vi "BonOMM-SAOMM.vi"() -> ()   [LabVIEW 2019] (continued)
                          frame False {
                            w3634 = i16 0 items=["tel coords", "tel offset", "guidage"] ("options")
                            n5502 = local read "Obslib"() -> (w3635:string[][])
                            n5503 = Build Array(w3632, w3631, w3630, w3629) -> (w3636:string[])
                            n5504 = call "Coords to chart(new).vi"("DataLine"=w3636, "options"=w3634, "Tableau entrant"=w3635) -> ("historique"=w3637:string[][])
                            n5505 = local write "Obslib"(w3637) -> ()
                          }
                          frame True {
                            w3643 = i16 0 items=["tel coords", "tel offset", "guidage"] ("options")
                            n5506 = local read "Obslib"() -> (w3644:string[][])
                            n5507 = Build Array(w3639, w3640, w3641, w3638) -> (w3645:string[])
                            n5508 = call "Coords to chart(new).vi"("DataLine"=w3645, "options"=w3643, "Tableau entrant"=w3644) -> ("historique"=w3646:string[][])
                            n5509 = local write "Obslib"(w3646) -> ()
                          }
                        }
                        "From library" <- w3626
                        n5510 = Number To Fractional String(number=w3599, width (-)=i16 4, precision (6)=w3619) -> (F-format string=w3612:string)  [unwired: 1 in]
                        n5511 = Number To Fractional String(number=w3598, width (-)=w3618, precision (6)=w3619) -> (F-format string=w3617:string)  [unwired: 1 in]
                        n5512 = Number To Fractional String(number=w3597, width (-)=w3618, precision (6)=w3619) -> (F-format string=w3616:string)  [unwired: 1 in]
                        n5513 = Search and Replace String(replace all?=w3613, input string=w3617, search string=w3614, replace string=w3615) -> (result string=w3611:string)  [unwired: 4 in, 3 out]
                        n5514 = Search and Replace String(replace all?=w3613, input string=w3616, search string=w3614, replace string=w3615) -> (result string=w3610:string)  [unwired: 4 in, 3 out]
                        n5515 = local read "path_pointing"() -> (w3609:path)
                        n5516 = Concatenate Strings(w3612, w3607, w3611, w3607, w3610, ".pnt") -> (w3608:string)
                        n5517 = Build Path(base path=w3609, name or relative path=w3608) -> (appended path=w3594:path)
                        n5518 = local read "File I/O Error"() -> (w3596:errorcluster)
                        n5519 = call "PNT-Data-Write.vi"("Path IN"=w3594, "Data Line"=w3593, "Error IN"=w3596) -> ("Error OUT"=w3595:errorcluster)  [unwired: 11 in, 1 out]
                        n5520 = local write "File I/O Error"(w3595) -> ()
                      }
                    }
                  }
                  frame True {
                    w3647 = 2
                    # "Début d'un déplacement"
                    # "Désactiver les boutons de TCS"
                    n5521 = property on="GO" class="Bool (strict)"("Disabled"=w3647) -> ()  [unwired: 2 in, 2 out]
                    n5522 = property on="ModifFoyer" class="Bool (strict)"("Disabled"=w3647) -> ()  [unwired: 2 in, 2 out]
                    n5523 = property on="Écran" class="Bool (strict)"("Disabled"=w3647) -> ()  [unwired: 2 in, 2 out]
                    n5524 = property on="ModCoor" class="Bool (strict)"("Disabled"=w3647) -> ()  [unwired: 2 in, 2 out]
                    n5525 = property on="Zénith" class="Bool (strict)"("Disabled"=w3647) -> ()  [unwired: 2 in, 2 out]
                    n5526 = property on="Range" class="Bool (strict)"("Disabled"=w3647) -> ()  [unwired: 2 in, 2 out]
                    n5527 = property on="Synctel" class="Bool (strict)"("Disabled"=w3647) -> ()  [unwired: 2 in, 2 out]
                    n5528 = property on="ModifRotation" class="Bool (strict)"("Disabled"=w3647) -> ()  [unwired: 2 in, 2 out]
                    n5529 = property on="Offset OK" class="Bool (strict)"("Disabled"=w3647) -> ()  [unwired: 2 in, 2 out]
                    n5530 = property on="ModifDome" class="Bool (strict)"("Disabled"=w3647) -> ()  [unwired: 2 in, 2 out]
                  }
                }
              }
            }
            n5531 = local read "Quit"() -> (w3405:bool)
          }
          "Événements Software" <- w978
          n5532 = while {
            tunnel: [w1297] -> w976
            stop <- w1297 stop-if-true
            # "Boucle périodique pour PrAMS + Hexapode + LVDTs\nÉvénements lents ..."
            n5533 = stacked-sequence {
              frame #0 {
                n5534 = disable-structure shown="Disabled" {
                  frame Disabled {
                    n5535 = local read "LVDT-RA"() -> (w1301:refnum<k21>)
                    n5536 = local read "LVDT Error"() -> (w1300:errorcluster)
                    n5537 = Unbundle By Name(w1300) -> ("status"=w1299:bool)
                    n5538 = case shown="Faux" w1299 {
                      tunnel: w1301 -> [w1314 _]
                      tunnel: w1300 -> [_ _]
                      frame False {
                        n5539 = call "Read-LVDT-Data.vi"("shared variable refnum"=w1314, "MaxLen"=631 ("timeout ms"), "Data IN"="LVDT-RA-Data") -> ("Graph Data"=w1308:dbl[], "Data OUT"=w1310:dbl[], "error out"=→"LVDT Error":errorcluster)  [unwired: 10 in]
                        "Graph Data" <- w1308
                        n5540 = local write "LVDT-RA-Data"(w1310) -> ()
                        n5541 = Subtract(x=w1308, y="LVDT-zero") -> (x-y=w1315:dbl[])
                        n5542 = Multiply(x="LVDT-scale", y=w1315) -> (x*y=w1305:dbl[])
                        n5543 = Array Size(array=w1305) -> (size(s)=w1304:i32)
                        n5544 = Decrement(x=w1304) -> (x-1=w1302:i32)
                        n5545 = Bundle(0.0, "LVDT-time"="LVDT-time", w1305) -> (→"LVDT-RA-coarse" →"LVDT-RA-closeup":cluster{dbl, "LVDT-time":dbl, dbl[]})  [unwired: 1 in]
                        n5546 = Index Array(array=w1305, index=w1302) -> (element=→"LVDT-RA-inst":dbl)
                      }
                      frame True {
                      }
                    }
                  }
                  frame Enabled {
                  }
                }
              }
              frame #1 {
                # "Si la communication avec TCS et PrAMS sont actives, on update les valeurs de ALT/AZ/ROT de Prams\n\nN.B. : L'erreur associée (#64) : est ignorée par la boucle \"emterror\" ci-bas ..."
                n5547 = local read "PrAMS COMM"() -> (w1319:bool)
                n5548 = local read "TCS COMM"() -> (w1320:bool)
                n5549 = And(x=w1320, y=w1319) -> (x .and. y?=w1318:bool)
                n5550 = case shown="Faux" w1318 {
                  frame False {
                  }
                  frame True {
                    n5551 = local read "Epoch Tel"() -> (w1334:dbl)
                    n5552 = local read "RA Tel"() -> (w1338:dbl)
                    n5553 = local read "DEC Tel"() -> (w1337:dbl)
                    n5554 = local read "AnnéeRL"() -> (w1333:dbl)
                    n5555 = local read "LST"() -> (w1332:dbl)
                    n5556 = call "ad2deg.vi"("DEC (sec)"=w1337, "RA (sec)"=w1338) -> ("DEC (°)"=w1335:dbl, "RA (°)"=w1336:dbl)
                    n5557 = call "ad2deg.vi"("RA (sec)"=w1332) -> ("RA (°)"=w1331:dbl)  [unwired: 1 in, 1 out]
                    n5558 = call "precess.vi"("Eq2"=w1333, "Eq1"=w1334, "DEC 1"=w1335, "RA 1"=w1336) -> ("DEC 2"=w1329:dbl, "RA 2"=w1339:dbl)
                    "DEC" <- w1329
                    n5559 = Subtract(x=w1331, y=w1339) -> (x-y=w1330:dbl)
                    "HA" <- w1330
                    n5560 = control-ref of="PrAMS-ACK"() -> (w1324:refnum<vi>)
                    n5561 = control-ref of="PrAMS actif"() -> (w1323:refnum<vi>)
                    n5562 = local read "PrAMS VRN"() -> (w1325:refnum<visa-resource-name>)
                    n5563 = local read "PrAMS Error"() -> (w1326:errorcluster)
                    n5564 = local read "Signature"() -> (w1328:u32)
                    n5565 = local read "MessageType"() -> (w1327:cluster{string[], u32[]})
                    n5566 = call "SAOMM-SetTelescopeProperties.vi"("PRAMMS-COMM IN"=w1325, "PramsActif"=w1323, "PrAMS-ACK"=w1324, "HA"=w1330, "DEC"=w1329, "Error IN"=w1326, "Signature"=w1328, "MsgTypeEnum"=w1327) -> ("PRAMMS-COMM OUT"=w1321:refnum<visa-resource-name>, "Error OUT"=w1322:errorcluster)  [unwired: 6 in]
                    n5567 = local write "PrAMS VRN"(w1321) -> ()
                    n5568 = local write "PrAMS Error"(w1322) -> ()
                  }
                }
              }
              frame #2 {
                # "L'angle ne peut être envoyé que si l'asservissement est OFF"
                n5569 = local read "Servo"() -> (w1340:bool)
                n5570 = case shown="Faux" w1340 {
                  frame False {
                    # "Prams à un 180° dans sa matrice d'Euler"
                    n5571 = local read "RotationEffective"() -> (w1351:dbl)
                    n5572 = control-ref of="PrAMS-ACK"() -> (w1343:refnum<vi>)
                    n5573 = local read "PrAMS VRN"() -> (w1346:refnum<visa-resource-name>)
                    n5574 = local read "PrAMS Error"() -> (w1347:errorcluster)
                    n5575 = local read "MessageType"() -> (w1348:cluster{string[], u32[]})
                    n5576 = control-ref of="PrAMS actif"() -> (w1344:refnum<vi>)
                    n5577 = local read "Signature"() -> (w1345:u32)
                    n5578 = call "Fix_angle.vi"("±180 -> 0-360?"=FALSE, "Angle IN"=w1351) -> ("Angle OUT"=w1350:dbl)  [unwired: 3 in]
                    n5579 = Negate(x=w1350) -> (-x=w1341:dbl)
                    n5580 = call-poly "SAOMM-Num2littleEndian.vi"("Number"=w1341) -> ("LiitleEndianedData"=w1349:u8[])  [unwired: 14 in]
                    n5581 = call "SAOMM-SendSET.vi"("PRAMMS-COMM IN"=w1346, "Active Refnum"=w1344, "PrAMS-ACK"=w1343, "Signature"=w1345, "Error IN"=w1347, "MessageType"=w1348, "Active SET"="emtSetMountingPlateAngle", "Value (little endianed byte array)"=w1349) -> ()  [unwired: 4 in, 4 out]
                  }
                  frame True {
                  }
                }
              }
              frame #3 {
                # "Enregistre environ 2 fois par \"Considered Lenght\""
                # "Update l'historique de guidage et enregistre log dans un fichier ..."
                n5582 = local read "Graph-Centroids"() -> (w1355:cluster{"TimeArray":dbl[], dbl[]}[])
                n5583 = Index Array(array=w1355) -> (element #1=w1372:cluster{"TimeArray":dbl[], dbl[]}, element #2=w1371:cluster{"TimeArray":dbl[], dbl[]})  [unwired: 2 in]
                n5584 = Unbundle(w1372) -> (w1369:dbl[])  [unwired: 1 out]
                n5585 = Unbundle(w1371) -> ("TimeArray"=w1354:dbl[], w1370:dbl[])
                n5586 = local read "LastSaveTimeStamp"() -> (w1361:dbl)
                n5587 = local read "ConsideredLenght"() -> (w1365:i32)
                n5588 = call "TimeStamp-Extractor.vi"("TimeStampArray"=w1354) -> ("LastTimestamp"=w1360:dbl)  [unwired: 12 in, 2 out]
                n5589 = To Double Precision Float(number=w1365) -> (double precision float=w1364:dbl)
                n5590 = call "Guide_error_histo.vi"("X Array"=w1369, "intervals"=11, "Y array"=w1370, "limite haute"=5.0, "limite basse"=-5.0 ("limite haute")) -> ("XY graph"=→"Guiderreur":cluster{dbl[], dbl[]}[])  [unwired: 1 out]
                n5591 = local read "CentroidsData"() -> (w1356:cluster{dbl[], dbl[]}[])
                n5592 = expression code="x/2"(w1364) -> (w1363:dbl)
                n5593 = Add(x=w1361, y=w1363) -> (x+y=w1362:dbl)
                n5594 = Greater?(x=w1360, y=w1362) -> (0:w1358:bool)
                n5595 = Or(x="ForceSaveToFile", y=w1358) -> (x .or. y?=w1359:bool)
                n5596 = case shown="Vrai" w1359 {
                  tunnel: w1360 -> [_ w1399]
                  tunnel: w1361 -> [_ w1384]
                  tunnel: w1356 -> [_ w1400]
                  frame False {
                  }
                  frame True {
                    # "Va peut-être perdre les quelques minutes juste avant la fermeture \n... pour ce que ça changera c'est beaucoup de travail."
                    n5597 = local read "path_trackfile"() -> (w1383:path)
                    n5598 = Strip Path(path=w1383) -> (stripped path=w1377:path)  [unwired: 1 out]
                    n5599 = local read "path_trackfile"() -> (w1397:path)
                    n5600 = Build Path(base path=w1377, name or relative path="Hexapod") -> (appended path=w1375:path)
                    n5601 = call "GetPathFromTimeStamp.vi"("UTC Time"=FALSE, "LocalTimeStamp"=w1384, "Changement de date à midi ?"=TRUE) -> ("Date String"=w1373:string)  [unwired: 11 in, 1 out]
                    n5602 = call "CheckAndCreateDirectory.vi"("Path IN"=w1375) -> ("Path OUT"=w1374:path, "Exists?"=w1380:bool, "Created?"=w1379:bool)  [unwired: 12 in]
                    n5603 = call "GetPathFromTimeStamp.vi"("UTC Time"=TRUE, "LocalTimeStamp"=w1399, "Changement de date à midi ?"=TRUE) -> ("Date String"=w1398:string)  [unwired: 11 in, 1 out]
                    n5604 = local read "ForceSaveToFile"() -> (w1389:bool)
                    n5605 = Build Path(base path=w1397, name or relative path=w1398) -> (appended path=w1396:path)
                    n5606 = Or(x=w1380, y=w1379) -> (x .or. y?=w1378:bool)
                    n5607 = local read "Servo"() -> (w1388:bool)
                    n5608 = case shown="Vrai" w1378 {
                      tunnel: w1384 -> [_ w1407]
                      tunnel: w1374 -> [_ w1406]
                      tunnel: w1373 -> [_ w1404]
                      frame False {
                      }
                      frame True {
                        # "Log de l'hexapode"
                        n5609 = Concatenate Strings(w1404, ".hex") -> (w1402:string)
                        n5610 = local read "HexXData"() -> (w1409:cluster{dbl[], dbl[]}[])
                        n5611 = local read "HexYData"() -> (w1408:cluster{dbl[], dbl[]}[])
                        n5612 = local read "CumulativeError"() -> (w1401:cluster{dbl[], dbl[]}[])
                        n5613 = Build Path(base path=w1406, name or relative path=w1402) -> (appended path=w1405:path)
                        n5614 = call "LogHexapodData.vi"("LogFilePath"=w1405, "TimeStampTreshold"=w1407, "X IN"=w1409, "Y IN"=w1408, "Cumul IN"=w1401) -> ()  [unwired: 10 in, 1 out]
                      }
                    }
                    n5615 = call "CheckAndCreateDirectory.vi"("Path IN"=w1396) -> ("Path OUT"=w1393:path, "Exists?"=w1395:bool, "Created?"=w1394:bool)  [unwired: 12 in]
                    n5616 = Or(x=w1395, y=w1394) -> (x .or. y?=w1391:bool)
                    n5617 = Or(x=w1388, y=w1389) -> (x .or. y?=w1387:bool)
                    n5618 = local read "TrackLogFilename"() -> (w1392:string)
                    n5619 = And(x=w1391, y=w1387) -> (x .and. y?=w1390:bool)
                    n5620 = case shown="Vrai" w1390 {
                      tunnel: w1400 -> [_ w1419]
                      tunnel: w1384 -> [_ w1416]
                      tunnel: w1393 -> [_ w1415]
                      tunnel: w1392 -> [_ w1413]
                      frame False {
                      }
                      frame True {
                        # "Log de guidage"
                        n5621 = local read "SNRData"() -> (w1411:cluster{dbl[], dbl[]}[])
                        n5622 = local read "FluxData"() -> (w1410:cluster{dbl[], dbl[]}[])
                        n5623 = Build Path(base path=w1415, name or relative path=w1413) -> (appended path=w1414:path)
                        n5624 = local write "ForceSaveToFile"(FALSE ("ForceSaveToFile")) -> ()
                        n5625 = local read "Dec Sonde"() -> (w1418:dbl)
                        n5626 = local read "RA Sonde"() -> (w1417:dbl)
                        n5627 = call "LogSourceData.vi"("LogFilePath"=w1414, "DECsonde"=w1418, "RAsonde"=w1417, "TimeStampTreshold"=w1416, "SNR IN"=w1411, "Flux IN"=w1410, "Centroids IN"=w1419) -> ()  [unwired: 8 in, 1 out]
                      }
                    }
                    "LastSaveTimeStamp" <- w1399
                  }
                }
              }
              frame #4 {
                n5628 = local read "LastProcID"() -> (w1431:u64)
                n5629 = local read "LastProcSavedID"() -> (w1432:u64)
                n5630 = Get Date/Time In Seconds() -> (seconds since 1Jan1904=w1423:timestamp)
                n5631 = local read "FalconProcTimeStamp"() -> (w1426:dbl)
                n5632 = local read "ConsideredLenght"() -> (w1427:i32)
                n5633 = To Double Precision Float(number=w1423) -> (double precision float=w1422:dbl)
                n5634 = Greater?(x=w1431, y=w1432) -> (0:w1430:bool)
                n5635 = To Double Precision Float(number=w1427) -> (double precision float=w1428:dbl)
                n5636 = Add(x=w1426, y=w1428) -> (x+y=w1425:dbl)
                n5637 = Greater?(x=w1422, y=w1425) -> (0:w1424:bool)
                n5638 = And(x=w1430, y=w1424) -> (x .and. y?=w1420:bool)
                n5639 = Or(x="SaveFalconProc", y=w1420) -> (x .or. y?=w1429:bool)
                n5640 = case shown="Vrai" w1429 {
                  tunnel: w1431 -> [_ w1434]
                  tunnel: w1422 -> [_ w1433]
                  frame False {
                  }
                  frame True {
                    # "Demande d'enregistre de la prochaine trame FalconProcessed"
                    n5641 = local read "path_data"() -> (w1438:path)
                    n5642 = local read "FalconProcData"() -> (w1435:u8[])
                    n5643 = local write "SaveFalconProc"(FALSE ("SaveFalconProc")) -> ()
                    n5644 = Build Path(base path=w1438, name or relative path="FalconProcessed") -> (appended path=w1436:path)
                    n5645 = call "WriteFalconProcessed.vi"("Path:~\\syslogs\\FalconProcessed"=w1436, "FalconProcessedData"=w1435) -> ()  [unwired: 13 in, 1 out]
                    "LastProcSavedID" <- w1434
                    "FalconProcTimeStamp" <- w1433
                  }
                }
              }
            }
            n5646 = Wait Until Next ms Multiple(millisecond multiple=u32 1000) -> ()  [unwired: 1 out]
            n5647 = local read "Quit"() -> (w1297:bool)
          }
          "Archivage SAOMM" <- w976
          n5648 = while {
            tunnel: [w2644] -> w971
            stop <- w2644 stop-if-true
            # "Boucle de gestions des clients et des commandes SÉRIE et TCP/IP"
            n5649 = stacked-sequence {
              frame #0 {
                # "Vérifie les demandes de connexions en déconnectant :\n  - celles qui sont inactives depuis plus d'une heure\n  x celles dont le client est le même (ne retient que la plus récente)\n  x celles ne provenant pas de 132.204.xxx.xxx"
                n5650 = String To IP(1:"Address du serveur") -> (0:w2651:u32)
                n5651 = call <vilib>:"TCP Listen.vi"("resolve remote address (T)"=FALSE, "net address"=w2651, "timeout ms (wait forever: -1)"=10, "port"="Port Local") -> ("error out"=w2646:errorcluster, "remote port"=w2649:u16, "remote address"=w2647:string, "connection ID"=w2648:refnum<k5>)  [unwired: 3 in, 1 out]
                n5652 = Not Equal?(x=w2647, y="") -> (x != y?=w2650:bool)
                n5653 = case shown="Vrai" w2650 {
                  tunnel: w2649 -> [_ w2658]
                  tunnel: w2648 -> [_ w2661]
                  tunnel: w2647 -> [_ w2657]
                  frame False {
                  }
                  frame True {
                    # "Ne conserve que l'adresse"
                    n5654 = local read "Clients"() -> (w2660:string[])
                    n5655 = for {
                      tunnel: w2660 -> [w2665] mode=indexing
                      tunnel: [w2664] -> w2659 mode=indexing
                      n5656 = Search/Split String(string=w2665, search string/char (-)=":") -> (substring before match=w2664:string)  [unwired: 1 in, 2 out]
                    }
                    n5657 = Search 1D Array(1D array=w2659, element=w2657) -> (index of element=w2656:i32)  [unwired: 1 in]
                    n5658 = Less Than 0?(x=w2656) -> (x < 0?=w2662:bool)
                    n5659 = case shown="Faux" w2662 {
                      tunnel: w2660 -> [w2678 w2702]
                      tunnel: w2661 -> [w2680 w2693]
                      tunnel: w2658 -> [w2679 w2705]
                      tunnel: w2657 -> [w2667 w2701]
                      tunnel: w2656 -> [_ w2695]
                      frame True {
                        # "l'adresse n'existe pas encore ..."
                        n5660 = Spreadsheet String To Array(delimiter (Tab)=".", format string="%s", spreadsheet string=w2667, array type (2D Dbl)=string[] []) -> (array=w2676:string[])
                        n5661 = Index Array(array=w2676) -> (element #1=w2674:string, element #2=w2673:string)  [unwired: 2 in]
                        n5662 = Equal?(x="132", y=w2674) -> (x = y?=w2670:bool)
                        n5663 = Equal?(x=w2673, y="204" ("x")) -> (x = y?=w2669:bool)
                        n5664 = And(x=w2670, y=w2669) -> (x .and. y?=w2668:bool)
                        n5665 = case shown="Vrai" w2668 {
                          tunnel: w2680 -> [w2682 w2692]
                          tunnel: w2679 -> [_ w2688]
                          tunnel: w2678 -> [_ w2685]
                          tunnel: w2667 -> [_ w2683]
                          frame False {
                            n5666 = TCP Close Connection(connection ID=w2682) -> (error out=w2681:errorcluster)  [unwired: 2 in, 1 out]
                            n5667 = local write "TCP/IP Error"(w2681) -> ()
                          }
                          frame True {
                            n5668 = local read "Clients ID"() -> (w2691:refnum<k5>[])
                            n5669 = Number To Decimal String(number=w2688) -> (decimal integer string=w2687:string)  [unwired: 1 in]
                            n5670 = Insert Into Array(array=w2691, new element=w2692) -> (→"Clients ID":refnum<k5>[])  [unwired: 1 in]
                            n5671 = Concatenate Strings(w2683, ":" ("string"), w2687) -> (w2686:string)
                            n5672 = Insert Into Array(array=w2685, new element=w2686) -> (→"Clients":string[])  [unwired: 1 in]
                          }
                        }
                      }
                      frame False {
                        n5673 = local read "Clients ID"() -> (w2696:refnum<k5>[])
                        n5674 = Number To Decimal String(number=w2705) -> (decimal integer string=w2704:string)  [unwired: 1 in]
                        n5675 = Index Array(array=w2696, index=w2695) -> (element=w2694:refnum<k5>)
                        n5676 = Concatenate Strings(w2701, ":" ("string"), w2704) -> (w2703:string)
                        n5677 = TCP Close Connection(connection ID=w2694) -> (error out=w2698:errorcluster)  [unwired: 2 in, 1 out]
                        n5678 = Replace Array Subset(array=w2702, new element=w2703, index=w2695) -> (w2697:string[])
                        n5679 = local write "TCP/IP Error"(w2698) -> ()
                        n5680 = local write "Clients"(w2697) -> ()
                        n5681 = Replace Array Subset(array=w2696, new element=w2693, index=w2695) -> (w2699:refnum<k5>[])
                        n5682 = local write "Clients ID"(w2699) -> ()
                      }
                    }
                  }
                }
                n5683 = local write "TCP/IP Error"(w2646) -> ()
              }
              frame #1 {
                # "Prends quelques millisecondes pour ramasser des commandes sur les ports ..."
                n5684 = flat-sequence {
                  frame #0 {
                    n5685 = control-ref of="FIFO actif"() -> (w2706:refnum<vi>)
                    n5686 = call "Fifo-Wait4Flag.vi"("Raise Flag ?"=TRUE, "Ctl Refnum IN"=w2706) -> ()  [unwired: 8 in, 2 out]
                  }
                  frame #1 {
                    # "Délai de réception pour chaque client (ms)"
                    n5687 = local read "Excmd VRN"() -> (w2716:refnum<visa-resource-name>)
                    n5688 = local read "TCP/IP Error"() -> (w2715:errorcluster)
                    n5689 = local read "Excom Error"() -> (w2708:errorcluster)
                    n5690 = local read "Clients ID"() -> (w2713:refnum<k5>[])
                    n5691 = local read "CmdFIFO"() -> (w2712:T14)
                    n5692 = call "WaitForCMD.vi"("Clients ID IN"=w2713, "Cmd FIFO IN"=w2712, "TCP/IP Error IN"=w2715, "Excmd VRN"=w2716, "Serial Error IN"=w2708, "Timeout"=u32 20) -> ("Cmd FIFO OUT"=→"CmdFIFO":T62, "TCP/IP Error"=w2714:errorcluster, "Serial Error"=w2709:errorcluster)  [unwired: 7 in]
                    n5693 = local write "TCP/IP Error"(w2714) -> ()
                    n5694 = local write "Excom Error"(w2709) -> ()
                  }
                  frame #2 {
                    n5695 = local write "FIFO actif"(FALSE) -> ()
                  }
                }
              }
            }
            n5696 = local read "Quit"() -> (w2644:bool)
          }
          "Scripts Listener" <- w971
          n5697 = while {
            tunnel: [w2718] -> w972
            stop <- w2718 stop-if-true
            # "Boucle pour la gestion des pop-up et autres événements non-synchronisés"
            n5698 = Array Size(array="FIFO d'erreur") -> (size(s)=w2722:i32)
            n5699 = Greater Than 0?(x=w2722) -> (x > 0?=w2721:bool)
            n5700 = case shown="Vrai" w2721 {
              tunnel: "FIFO d'erreur" -> [_ w2725]
              frame False {
              }
              frame True {
                n5701 = Delete From Array(array=w2725, length=1, index=0) -> (deleted portion=w2726:T7, array with subset deleted=w2724:T7)
                n5702 = local write "FIFO d'erreur"(w2724) -> ()
                n5703 = Index Array(array=w2726) -> (element=w2723:T63)  [unwired: 1 in]
                n5704 = Unbundle By Name(w2723) -> ("Source"=w2729:string)
                n5705 = case shown="\"offset\"" w2729 {
                  tunnel: w2723 -> [w2730 w2733 w2734 w2736 w2738 _]
                  frame "PrAMS" {
                    n5706 = Unbundle By Name(w2730) -> ("Comment"=w2731:string)
                    n5707 = One Button Dialog(message=w2731) -> ()  [unwired: 1 in, 1 out]
                  }
                  frame "Hexapod" {
                    n5708 = Unbundle By Name(w2733) -> ("Comment"=w2732:string)
                    n5709 = One Button Dialog(message=w2732) -> ()  [unwired: 1 in, 1 out]
                  }
                  frame "offset" {
                    # "Error Code\nb0 : 01 : Erreur mineure\nb1 : 02 : Intervention nécessaire\nb2 : 04 : Erreur avec TCS\nb3 : 08 : Erreur avec Tables\nb4 : 16 : Erreur avec MaximDL\nb5 : 32 : Erreur avec Périphérique\nb6 : 64 : Erreur Majeure\nb7 : 128 : Commande inexistante"
                    # "Warning Code\nb0 : 01 : Micro-Offset non effecuté (pas de guidage)\nb1 : 02 : Guidage non-redémarré, référence perdue\nb2 : 04 : Erreur avec TCS\nb3 : 08 : Erreur avec Tables\nb4 : 16 : Erreur MaximDL/Caméra de guidage\nb5 : 32 : \nb6 : 64 : Erreur avec la base de données USNO\nb7 : 128 : Impossible d'arrêter le télescope ou les tables de guidages !!!"
                    n5710 = call "Offset_Error&Warnings.vi"("Cluster"=w2734) -> ()  [unwired: 6 in]
                  }
                  frame "ETCS" {
                    # "Écrit le commentaire directement dans le dialog"
                    n5711 = Unbundle By Name(w2736) -> ("Comment"=w2735:string)
                    n5712 = One Button Dialog(message=w2735) -> ()  [unwired: 1 in, 1 out]
                  }
                  frame "TCS" {
                    n5713 = Unbundle By Name(w2738) -> ("Comment"=w2737:string)
                    n5714 = One Button Dialog(message=w2737) -> ()  [unwired: 1 in, 1 out]
                  }
                  frame Default {
                    # "Source de l'erreur indéfinie ..."
                  }
                }
              }
            }
            n5715 = Wait (ms)(milliseconds to wait=u32 50) -> ()  [unwired: 1 out]
            n5716 = local read "Quit"() -> (w2718:bool)
          }
          "Afficahge d'erreur" <- w972
          n5717 = while {
            tunnel: w983 -> [w1056]
            tunnel: [w1052] -> w973
            stop <- w1052 stop-if-true
            # "ms to wait for 1st 4 bytes"
            n5718 = local read "Signature"() -> (w1061:u32)
            n5719 = local read "PrAMS Error"() -> (w1058:errorcluster)
            n5720 = local read "Hexapod VRN"() -> (w1057:refnum<visa-resource-name>)
            n5721 = local read "MessageType"() -> (w1059:cluster{string[], u32[]})
            n5722 = call "PRAMMS-LISTENER.vi"("PRAMMS-COMM IN"=w1057, "Bool Refnum"=w1056, "MessageTypeArray"=w1059, "Signature"=w1061, "Error IN"=w1058, "ReadTimeOut"=5) -> ("Type"=w1054:string, "ByteArray"=w1053:u8[], "Received?"=w1055:bool)  [unwired: 4 in, 3 out]
            n5723 = case shown="Vrai" w1055 {
              tunnel: w1054 -> [_ w1063]
              tunnel: w1053 -> [_ w1062]
              frame False {
              }
              frame True {
                n5724 = case shown="\"emtAcknowledgment\"" w1063 {
                  selector: w1063 -> [w1065 _ _ w1094 _ _ w1116 _ _ _]
                  tunnel: w1062 -> [w1064 w1081 _ w1093 w1114 _ w1117 _ _ w1168]
                  frame Default {
                    n5725 = Type Cast(x=w1064) -> (*(type *) &x=w1069:string)  [unwired: 1 in]
                    n5726 = local read "Dump"() -> (w1066:string)
                    n5727 = Concatenate Strings(w1066, w1065, " : " ("string"), w1069, "\r") -> (w1070:string)
                    n5728 = local read "nDumped"() -> (w1072:i32)
                    n5729 = Increment(x=w1072) -> (x+1=→"nDumped":i32)
                    n5730 = local write "Dump"(w1070) -> ()
                  }
                  frame "emtError" {
                    # "Rempli le fifo d'erreur"
                    # "Si un code d'erreur est retourné, il sera mis négatif et entrez dans la variable ACK"
                    n5731 = To Unsigned Long Integer(number=u32 0) -> (unsigned 32bit integer=w1079:u32)
                    n5732 = call-poly "SAOMM-EXTRACT-DATA.vi"("UINT32"=w1079, "Data"=w1081) -> ("Value"=w1076:u32)  [unwired: 10 in, 3 out]
                    n5733 = Negate(x=1) -> (-x=w1073:i32)
                    n5734 = Not Equal To 0?(x=w1076) -> (x != 0?=w1077:bool)
                    n5735 = local write "Hexapod-ACK"(w1073) -> ()
                    n5736 = case shown="Faux" w1077 {
                      tunnel: w1076 -> [_ w1089]
                      tunnel: ["Erreur reçu de l'Hexapode (code : indéfini)" w1085] -> w1075
                      frame False {
                      }
                      frame True {
                        n5737 = Number To Decimal String(number=w1089) -> (decimal integer string=w1088:string)  [unwired: 1 in]
                        n5738 = Concatenate Strings("Erreur reçu de l'Hexapode (code : ", w1088, ")") -> (w1085:string)
                      }
                    }
                    n5739 = local read "FIFO d'erreur"() -> (w1083:T7)
                    n5740 = call "Error_Format.vi"("FIFO IN"=w1083, "Error Code IN"=w1076, "Source"="Hexapod", "Comment"=w1075) -> ("FIFO OUT"=w1082:T7)  [unwired: 13 in, 2 out]
                    n5741 = local write "FIFO d'erreur"(w1082) -> ()
                  }
                  frame "emtAcknowledgment" {
                    n5742 = local read "Nb_ACK (hex)"() -> (w1091:i32)
                    n5743 = Increment(x=w1091) -> (x+1=→"Nb_ACK (hex)":i32)
                    "Hexapod-ACK" <- 1
                  }
                  frame "emtUAxis", "emtVAxis", "emtWAxis", "emtXAxis", "emtYAxis", "emtZAxis" {
                    n5744 = To Double Precision Float(number=0.0) -> (double precision float=w1096:dbl)
                    n5745 = call-poly "SAOMM-EXTRACT-DATA.vi"("DBL"=w1096, "Data"=w1093) -> ("Value"=w1097:dbl)  [unwired: 10 in, 3 out]
                    n5746 = case shown="\"emtWAxis\"" w1094 {
                      selector: w1094 -> [w1099 _ _ _ _ _ _]
                      tunnel: w1097 -> [w1102 w1105 w1106 w1107 w1108 w1109 w1110]
                      frame Default {
                        w1101 = "\r"
                        n5747 = Type Cast(type=w1101, x=w1102) -> (*(type *) &x=w1103:string)
                        n5748 = local read "Dump"() -> (w1098:string)
                        n5749 = Concatenate Strings(w1098, w1099, " : " ("string"), w1103, w1101) -> (w1104:string)
                        n5750 = local write "Dump"(w1104) -> ()
                      }
                      frame "emtXAxis" {
                        n5751 = local write "HexX"(w1105) -> ()
                      }
                      frame "emtYAxis" {
                        n5752 = local write "HexY"(w1106) -> ()
                      }
                      frame "emtZAxis" {
                        n5753 = local write "HexZ"(w1107) -> ()
                      }
                      frame "emtUAxis" {
                        n5754 = local write "HexU"(w1108) -> ()
                      }
                      frame "emtVAxis" {
                        n5755 = local write "HexV"(w1109) -> ()
                      }
                      frame "emtWAxis" {
                        n5756 = local write "HexW"(w1110) -> ()
                      }
                    }
                  }
                  frame "emtVelocity" {
                    n5757 = To Double Precision Float(number=0.0) -> (double precision float=w1112:dbl)
                    n5758 = call-poly "SAOMM-EXTRACT-DATA.vi"("DBL"=w1112, "Data"=w1114) -> ("Value"=w1111:dbl)  [unwired: 10 in, 3 out]
                    n5759 = local write "Vitesse [mm/s]"(w1111) -> ()
                  }
                  frame "emtMoveIncrement" {
                    # "Quel format cela aura-t-il"
                  }
                  frame "emtUAxisOffset", "emtVAxisOffset", "emtWAxisOffset", "emtXAxisOffset", "emtYAxisOffset", "emtZAxisOffset" {
                    n5760 = To Double Precision Float(number=0.0) -> (double precision float=w1119:dbl)
                    n5761 = call-poly "SAOMM-EXTRACT-DATA.vi"("DBL"=w1119, "Data"=w1117) -> ("Value"=w1115:dbl)  [unwired: 10 in, 3 out]
                    n5762 = case shown="\"emtWAxisOffset\"" w1116 {
                      selector: w1116 -> [w1121 _ _ _ _ _ _]
                      tunnel: w1115 -> [w1120 w1127 w1128 w1129 w1130 w1131 w1132]
                      frame Default {
                        w1124 = "\r"
                        n5763 = Type Cast(type=w1124, x=w1120) -> (*(type *) &x=w1125:string)
                        n5764 = local read "Dump"() -> (w1122:string)
                        n5765 = Concatenate Strings(w1122, w1121, " : " ("string"), w1125, w1124) -> (w1126:string)
                        n5766 = local write "Dump"(w1126) -> ()
                      }
                      frame "emtXAxisOffset" {
                        n5767 = local write "Offset X"(w1127) -> ()
                      }
                      frame "emtYAxisOffset" {
                        n5768 = local write "Offset Y"(w1128) -> ()
                      }
                      frame "emtZAxisOffset" {
                        n5769 = local write "Offset Z"(w1129) -> ()
                      }
                      frame "emtUAxisOffset" {
                        n5770 = local write "Offset U"(w1130) -> ()
                      }
                      frame "emtVAxisOffset" {
                        n5771 = local write "Offset V"(w1131) -> ()
                      }
                      frame "emtWAxisOffset" {
                        n5772 = flat-sequence {
                          tunnel: w1132 -> [w1133]
                          frame #0 {
                            n5773 = local write "Offset W"(w1133) -> ()
                          }
                          frame #1 {
                            n5774 = local read "HexapodQuery"() -> (w1135:u32)
                            n5775 = Tick Count (ms)() -> (millisecond timer value=w1136:u32)
                            n5776 = local write "QueryingHexapod"(FALSE ("QueryingHexapod")) -> ()
                            n5777 = Subtract(x=w1136, y=w1135) -> (x-y=w1134:u32)
                            n5778 = local write "HexapodQuery"(w1134) -> ()
                          }
                        }
                      }
                    }
                  }
                  frame "emtMoveStarted" {
                    n5779 = local write "HxMoving"(TRUE) -> ()
                  }
                  frame "emtMoveStopped" {
                    n5780 = local write "HxMoving"(FALSE) -> ()
                  }
                  frame "emtMoving" {
                    w1149 = 0.0
                    w1150 = u8[] []
                    # "emtMoving\n\nTimeStamp(U64)\nXAxis(DBL)\nYAxis(DBL)\nZAxis(DBL)\nUAxis(DBL)\nZAxis(DBL)"
                    n5781 = Type Cast(type=dbl[] [], x=w1168) -> (*(type *) &x=w1166:dbl[])
                    n5782 = Index Array(array=w1166) -> (element #1=w1165:dbl, element #2=w1162:dbl, element #3=w1148:dbl, element #4=w1147:dbl, element #5=w1146:dbl, element #6=w1145:dbl)  [unwired: 6 in]
                    n5783 = To Unsigned Quad Integer(1:u64 0) -> (0:w1164:u64)
                    n5784 = Type Cast(type=w1164, x=w1165) -> (*(type *) &x=→"QueryTimeStamp":u64)
                    n5785 = Type Cast(type=w1150, x=w1147) -> (*(type *) &x=w1156:u8[])
                    n5786 = Type Cast(type=w1150, x=w1146) -> (*(type *) &x=w1153:u8[])
                    n5787 = Type Cast(type=w1150, x=w1145) -> (*(type *) &x=w1152:u8[])
                    n5788 = Type Cast(type=w1150, x=w1162) -> (*(type *) &x=w1161:u8[])
                    n5789 = Type Cast(type=w1150, x=w1148) -> (*(type *) &x=w1157:u8[])
                    n5790 = Reverse 1D Array(array=w1161) -> (reversed array=w1160:u8[])
                    n5791 = Reverse 1D Array(array=w1157) -> (reversed array=w1158:u8[])
                    n5792 = Reverse 1D Array(array=w1156) -> (reversed array=w1155:u8[])
                    n5793 = Reverse 1D Array(array=w1153) -> (reversed array=w1154:u8[])
                    n5794 = Reverse 1D Array(array=w1152) -> (reversed array=w1151:u8[])
                    n5795 = Type Cast(type=w1149, x=w1155) -> (*(type *) &x=w1143:dbl)
                    n5796 = Type Cast(type=w1149, x=w1154) -> (*(type *) &x=w1142:dbl)
                    n5797 = Type Cast(type=w1149, x=w1151) -> (*(type *) &x=w1141:dbl)
                    n5798 = Type Cast(type=w1149, x=w1160) -> (*(type *) &x=w1159:dbl)
                    n5799 = Type Cast(type=w1149, x=w1158) -> (*(type *) &x=w1144:dbl)
                    n5800 = local write "HexX"(w1159) -> ()
                    n5801 = local write "HexY"(w1144) -> ()
                    n5802 = local write "HexZ"(w1143) -> ()
                    n5803 = local write "HexU"(w1142) -> ()
                    n5804 = local write "HexV"(w1141) -> ()
                  }
                }
              }
            }
            n5805 = local read "Quit"() -> (w1052:bool)
          }
          "Hexapod Listener" <- w973
          n5806 = while {
            tunnel: [w4128] -> w981
            stop <- w4128 stop-if-true
            # "Structure de gestion des événements prioritaires"
            n5807 = event shown="[1] \"stoptable\": Valeur changée" {
              selector: _ -> [_ _ _ _]
              dyn-events: _ -> [_ _ _ _]
              timeout: 250 -> [_ _ _ _]
              event Timeout {
                n5808 = event-data() -> ()  [unwired: 1 in, 1 out]
              }
              event "stoptable": Value Change {
                n5809 = event-data() -> ("NewVal"=w4130:bool)  [unwired: 1 in, 4 out]
                n5810 = case shown="Vrai" w4130 {
                  frame False {
                  }
                  frame True {
                    n5811 = flat-sequence {
                      frame #0 {
                        w4131 = FALSE ("stoptable")
                        n5812 = local read "Table VRN"() -> (w4141:refnum<visa-resource-name>)
                        n5813 = local write "CorrectZ"(w4131) -> ()
                        n5814 = local write "CorrectXY"(w4131) -> ()
                        n5815 = local write "CurvCorrect"(w4131) -> ()
                        n5816 = local write "Focusing"(w4131) -> ()
                        n5817 = local write "stoptable"(w4131) -> ()
                        n5818 = control-ref of="Table actif"() -> (w4136:refnum<vi>)
                        n5819 = call "Newmark-Stop.vi"("Table VRN IN"=w4141, "Bool Refnum"=w4136) -> ("Table VRN OUT"=w4140:refnum<visa-resource-name>, "Error OUT"=w4139:errorcluster)  [unwired: 12 in]
                        n5820 = call "Newmark-Clear.vi"("Table VRN IN"=w4140, "Bool Refnum"=w4136, "Error IN"=w4139) -> ("Table VRN OUT"=w4138:refnum<visa-resource-name>, "Error OUT"=w4137:errorcluster)  [unwired: 11 in]
                        n5821 = control-ref of="TERMINAL"() -> (w4134:refnum<vi>)
                        n5822 = control-ref of="Indicateur d'état"() -> (w4135:refnum<vi>)
                        n5823 = local write "Table VRN"(w4138) -> ()
                        n5824 = local write "Table Error"(w4137) -> ()
                        n5825 = property on="Origine" class="Bool (strict)"("Blinking"=FALSE) -> ()  [unwired: 2 in, 2 out]
                        n5826 = call "TERMINAL.vi"("Indicateur Refnum"=w4135, "Terminal Refnum"=w4134, "Indicateur d'état"="Arrêt d'urgence des tables") -> ()
                      }
                      frame #1 {
                        # "Arrêt de l'initialisation des tables ..."
                        # "Wait for the stages to stop"
                        n5827 = while {
                          i -> [w4150]
                          stop <- w4151 stop-if-true
                          n5828 = local read "MovingXY"() -> (w4147:bool)
                          n5829 = Wait (ms)(milliseconds to wait=u32 250) -> ()  [unwired: 1 out]
                          n5830 = Greater?(x=w4150, y=5) -> (0:w4148:bool)
                          n5831 = Not(x=w4147) -> (.not. x?=w4146:bool)
                          n5832 = Or(x=w4146, y=w4148) -> (x .or. y?=w4151:bool)
                        }
                        n5833 = local read "Origine en cours..."() -> (w4142:bool)
                        n5834 = case shown="Vrai" w4142 {
                          selector: w4142 -> [_ w4143]
                          frame False {
                          }
                          frame True {
                            n5835 = while {
                              stop <- w4145 continue-if-true
                              n5836 = local read "Origine en cours..."() -> (w4145:bool)
                              n5837 = Wait (ms)(milliseconds to wait=u32 50) -> ()  [unwired: 1 out]
                            }
                            "Quit_Origine" <- w4143
                          }
                        }
                      }
                      frame #2 {
                        w4153 = FALSE
                        # "Remise à zéro des exceptions ..."
                        n5838 = flat-sequence {
                          frame #0 {
                            n5839 = control-ref of="Table actif"() -> (w4158:refnum<vi>)
                            n5840 = call "Newmark-Wait4Flag.vi"("Raise Flag ?"=TRUE, "Ctl Refnum IN"=w4158) -> ()  [unwired: 8 in, 2 out]
                          }
                          frame #1 {
                            n5841 = local write "Exceptions"(T3 {"Command Error"=FALSE, "Slip/Stall"=FALSE, "Overtravel"=FALSE, "Done"=FALSE, "nError"=0, "nSlip"=0, "nOT"=0, "nDone"=0} ("Exceptions")) -> ()
                          }
                          frame #2 {
                            n5842 = local write "Table actif"(FALSE ("Table actif")) -> ()
                          }
                        }
                        n5843 = local read "Position X"() -> (w4156:dbl)
                        n5844 = local read "Position Y"() -> (w4155:dbl)
                        n5845 = local read "Position Z"() -> (w4154:dbl)
                        n5846 = local write "Cible X"(w4156) -> ()
                        n5847 = local write "Cible Z"(w4154) -> ()
                        n5848 = local write "Cible Y"(w4155) -> ()
                        n5849 = local write "Calibration"(w4153) -> ()
                        n5850 = local write "Quit_Origine"(w4153) -> ()
                        n5851 = local write "RangeTable"(w4153) -> ()
                        n5852 = local write "Alacible"(w4153) -> ()
                        n5853 = local write "Origine"(w4153) -> ()
                        n5854 = local write "Centre"(w4153) -> ()
                      }
                    }
                  }
                }
              }
              event "StopTel": Value Change {
                # "Boucle de \nsurveillance du \nbouton STOP"
                n5855 = event-data() -> ("NewVal"=w4164:bool)  [unwired: 1 in, 4 out]
                n5856 = control-ref of="TERMINAL"() -> (w4162:refnum<vi>)
                n5857 = control-ref of="Indicateur d'état"() -> (w4163:refnum<vi>)
                n5858 = call "TERMINAL.vi"("Indicateur Refnum"=w4163, "Terminal Refnum"=w4162, "Indicateur d'état"="Appui du bouton \"STOP TÉL\"") -> ()
                n5859 = case shown="Vrai" w4164 {
                  frame False {
                  }
                  frame True {
                    n5860 = flat-sequence {
                      tunnel: [w4190] -> w4165
                      frame #0 {
                        w4167 = FALSE ("Blinking")
                        w4169 = 0
                        w4170 = 0
                        w4171 = FALSE
                        n5861 = local read "Focus slew"() -> (w4166:bool)
                        n5862 = property on="GO" class="Bool (strict)"("Disabled"=w4170) -> ()  [unwired: 2 in, 2 out]
                        n5863 = property on="Zénith" class="Bool (strict)"("Disabled"=w4170) -> ()  [unwired: 2 in, 2 out]
                        n5864 = property on="Range" class="Bool (strict)"("Disabled"=w4170) -> ()  [unwired: 2 in, 2 out]
                        n5865 = property on="Écran" class="Bool (strict)"("Disabled"=w4170) -> ()  [unwired: 2 in, 2 out]
                        n5866 = property on="ModifRotation" class="Bool (strict)"("Disabled"=w4170) -> ()  [unwired: 2 in, 2 out]
                        n5867 = property on="ModifDome" class="Bool (strict)"("Disabled"=w4170) -> ()  [unwired: 2 in, 2 out]
                        n5868 = property on="StopTel" class="Bool (strict)"("Disabled"=w4170) -> ()  [unwired: 2 in, 2 out]
                        n5869 = case shown="Vrai" w4166 {
                          frame False {
                          }
                          frame True {
                            "Annulation du foyer" <- TRUE
                          }
                        }
                        n5870 = local write "From library"(FALSE ("Déplacement usager")) -> ()
                        n5871 = property on="Offset OK" class="Bool (strict)"("Disabled"=w4169) -> ()  [unwired: 2 in, 2 out]
                        n5872 = property on="Coupole-Tél" class="Bool (strict)"("Disabled"=w4169) -> ()  [unwired: 2 in, 2 out]
                        n5873 = property on="ModCoor" class="Bool (strict)"("Disabled"=w4169) -> ()  [unwired: 2 in, 2 out]
                        n5874 = property on="ModifFoyer" class="Bool (strict)"("Disabled"=w4169) -> ()  [unwired: 2 in, 2 out]
                        n5875 = property on="Synctel" class="Bool (strict)"("Disabled"=w4169) -> ()  [unwired: 2 in, 2 out]
                        n5876 = local write "StopTel"(FALSE ("Raise Flag ?")) -> ()
                        n5877 = local write "Zénith"(w4171) -> ()
                        n5878 = local write "Écran"(w4171) -> ()
                        n5879 = local write "Range"(w4171) -> ()
                        n5880 = property on="ModifRotation" class="Bool (strict)"("Blinking"=w4167) -> ()  [unwired: 2 in, 2 out]
                        n5881 = property on="ModifDome" class="Bool (strict)"("Blinking"=w4167) -> ()  [unwired: 2 in, 2 out]
                        n5882 = property on="Zénith" class="Bool (strict)"("Blinking"=w4167) -> ()  [unwired: 2 in, 2 out]
                        n5883 = property on="Range" class="Bool (strict)"("Blinking"=w4167) -> ()  [unwired: 2 in, 2 out]
                        n5884 = property on="Écran" class="Bool (strict)"("Blinking"=w4167) -> ()  [unwired: 2 in, 2 out]
                        n5885 = property on="ModifFoyer" class="Bool (strict)"("Blinking"=w4167) -> ()  [unwired: 2 in, 2 out]
                      }
                      frame #1 {
                        n5886 = control-ref of="TCS actif"() -> (w4174:refnum<vi>)
                        n5887 = local read "TCS VRN"() -> (w4187:refnum<visa-resource-name>)
                        n5888 = call "EXCOM-CMD.vi"("VRN IN"=w4187, "Bool Refnum"=w4174, "Commande #"=13) -> ("VRN OUT"=w4188:refnum<visa-resource-name>, "OK Done"=w4190:bool, "Error OUT"=w4189:errorcluster)  [unwired: 10 in]
                        n5889 = call "EXCOM-28.vi"("VISA resource name"=w4188, "Error IN"=w4189, "Bool Refnum"=w4174) -> ("VISA resource name dup"=w4175:refnum<visa-resource-name>, "NORA"=w4184:dbl, "NODEC"=w4183:dbl, "Error OUT"=w4185:errorcluster)  [unwired: 11 in, 2 out]
                        n5890 = local read "NO epoch"() -> (w4182:dbl)
                        n5891 = local read "LST"() -> (w4180:dbl)
                        n5892 = local write "TCS Error"(w4185) -> ()
                        n5893 = local write "TCS VRN"(w4175) -> ()
                        n5894 = call "Object_properties.vi"("Target RA"=w4184, "Target DEC"=w4183, "Target Epoch"=w4182, "Sideral Time"=w4180) -> ("NO RA"=w4179:string, "NO DEC"=w4178:string, "NO Epoch"=w4181:dbl, "NO HA"=w4176:dbl, "NO AM"=w4177:dbl)  [unwired: 7 in]
                        n5895 = local write "NO epoch"(w4181) -> ()
                        n5896 = local write "N.O. Déc."(w4178) -> ()
                        n5897 = local write "N.O. A.D."(w4179) -> ()
                        n5898 = local write "NO AM"(w4177) -> ()
                        n5899 = local write "NO HA"(w4176) -> ()
                      }
                    }
                    n5900 = case shown="Faux" w4165 {
                      selector: w4165 -> [w4191 w4195]
                      frame False {
                        n5901 = local write "StopTel"(w4191) -> ()
                        n5902 = One Button Dialog(message="ATTENTION!!\nLa commande STOP a échoué.\nVérifiez TCS.", button name ("OK")="OK" ("nom du bouton (\"OK\")")) -> ()  [unwired: 1 out]
                      }
                      frame True {
                        n5903 = Not(x=w4195) -> (.not. x?=w4194:bool)
                        n5904 = local write "StopTel"(w4194) -> ()
                      }
                    }
                  }
                }
              }
              event "cancel-raf": Mouse Down {
                # "Pas certain que ça fasse quoique ce soit ?!?"
                n5905 = event-data() -> ()  [unwired: 1 in, 8 out]
                n5906 = case shown="Vrai" "cancel-raf" {
                  frame False {
                  }
                  frame True {
                    n5907 = local write "cancel-raf"(FALSE) -> ()
                    n5908 = control-ref of="TERMINAL"() -> (w4198:refnum<vi>)
                    n5909 = control-ref of="Indicateur d'état"() -> (w4199:refnum<vi>)
                    n5910 = call "TERMINAL.vi"("Indicateur Refnum"=w4199, "Terminal Refnum"=w4198, "Indicateur d'état"="Annulation du déplacement de la roue à filtre") -> ()
                    "Annulation en cours" <- TRUE
                  }
                }
              }
            }
            n5911 = local read "Quit"() -> (w4128:bool)
          }
          "Stops" <- w981
          n5912 = while {
            tunnel: [w2739] -> w980
            stop <- w2739 stop-if-true
            w2756 = 1.0
            # "Ajouté une condition sur l'état de la communication ?"
            # "Boucle de synchronisation avec StarryNight"
            n5913 = local read "AnnéeRL"() -> (w2740:dbl)
            n5914 = global read "Globals.vi" "ScopeSim._Telescope"() -> (w2752:refnum<k7>)
            n5915 = call "Get_SN_Coords.vi"("Output EPOCH"=w2740, "ScopeSim._Telescope"=w2752) -> ("DEC(sec)"=w2750:dbl, "RA(sec)"=w2751:dbl)  [unwired: 8 in]
            n5916 = local read "Dectmp"() -> (w2759:dbl)
            n5917 = local read "RAtmp"() -> (w2758:dbl)
            n5918 = Subtract(x=w2751, y=w2758) -> (x-y=w2757:dbl)
            n5919 = Subtract(x=w2759, y=w2750) -> (x-y=w2755:dbl)
            n5920 = Absolute Value(x=w2755) -> (abs(x)=w2753:dbl)
            n5921 = Absolute Value(x=w2757) -> (abs(x)=w2754:dbl)
            n5922 = Greater?(x=w2754, y=w2756) -> (0:w2749:bool)
            n5923 = Less Or Equal?(x=w2756, y=w2753) -> (x <= y?=w2746:bool)
            n5924 = Not Equal To 0?(x=w2751) -> (x != 0?=w2748:bool)
            n5925 = Not Equal To 0?(x=w2750) -> (x != 0?=w2745:bool)
            n5926 = And(x=w2748, y=w2749) -> (x .and. y?=w2747:bool)
            n5927 = And(x=w2746, y=w2745) -> (x .and. y?=w2744:bool)
            n5928 = Or(x=w2747, y=w2744) -> (x .or. y?=w2743:bool)
            n5929 = And(x="Sync_Ready", y=w2743) -> (x .and. y?=w2742:bool)
            n5930 = case shown="Vrai" w2742 {
              tunnel: w2751 -> [_ w2774]
              tunnel: w2750 -> [_ w2776]
              tunnel: "Sync_Ready" -> [_ _]
              tunnel: w2740 -> [_ w2771]
              frame False {
                n5931 = global read "Globals.vi" "ScopeSim._Telescope"() -> (w2766:refnum<k7>)
                n5932 = local read "Epoch Tel"() -> (w2765:dbl)
                n5933 = local read "RA Tel"() -> (w2763:dbl)
                n5934 = local read "DEC Tel"() -> (w2764:dbl)
                n5935 = call "Set_SN_Coords.vi"("Coords EPOCH"=w2765, "input_DEC"=w2764, "input_RA"=w2763, "ScopeSim._Telescope"=w2766) -> ("precessed_DEC"=w2761:dbl, "precessed_RA"=w2762:dbl)  [unwired: 6 in]
                n5936 = local write "Dectmp"(w2761) -> ()
                n5937 = local write "RAtmp"(w2762) -> ()
              }
              frame True {
                # "Affiche les coordonnées dans l'époque\nd'affichage du télescope pour que la\ncomparaison soit facile."
                # "Mode test en attendant ..."
                n5938 = local read "Epoch Tel"() -> (w2772:dbl)
                n5939 = local write "RAtmp"(w2774) -> ()
                n5940 = local read "LST"() -> (w2775:dbl)
                n5941 = local write "Dectmp"(w2776) -> ()
                n5942 = call "Object_properties.vi"("Target RA"=w2774, "Target DEC"=w2776, "Target Epoch"=w2772, "Sideral Time"=w2775) -> ("NO RA"=w2768:string, "NO DEC"=w2767:string, "NO Epoch"=w2773:dbl, "NO HA"=w2769:dbl, "NO AM"=w2770:dbl)  [unwired: 7 in]
                n5943 = call "Mode sync(pop-up).vi"("Époq. in"=w2773, "Déc. in"=w2767, "RA in"=w2768) -> ("Valeur"=w2777:u32)
                n5944 = case shown="2" w2777 {
                  tunnel: w2774 -> [w2789 _ w2821 w2842]
                  tunnel: w2776 -> [w2788 _ w2822 w2841]
                  tunnel: w2772 -> [_ _ w2813 _]
                  tunnel: w2771 -> [_ _ w2812 w2838]
                  tunnel: w2770 -> [_ _ _ w2839]
                  tunnel: w2769 -> [_ _ _ w2840]
                  tunnel: w2768 -> [_ _ _ w2837]
                  tunnel: w2767 -> [_ _ _ w2836]
                  frame 0, Default {
                    w2778 = u16 1 items=["Region d'intérêt", "Prévisualisation"] ("ImageUsage")
                    # "Vérifier si ça marche ..."
                    n5945 = local read "AnnéeRL"() -> (w2785:dbl)
                    n5946 = local read "Epoch Tel"() -> (w2784:dbl)
                    n5947 = call "ad2deg.vi"("DEC (sec)"=w2788, "RA (sec)"=w2789) -> ("DEC (°)"=w2790:dbl, "RA (°)"=w2791:dbl)
                    n5948 = call "precess.vi"("Eq2"=w2784, "Eq1"=w2785, "DEC 1"=w2790, "RA 1"=w2791) -> ("DEC 2"=w2787:dbl, "RA 2"=w2786:dbl)
                    n5949 = global write "Globals.vi" "RA Tmp"(w2786) -> ()
                    n5950 = global write "Globals.vi" "DEC Tmp"(w2787) -> ()
                    n5951 = local read "ImgAstrom"() -> (w2799:T4)
                    n5952 = local read "FieldAstrom"() -> (w2802:T4)
                    n5953 = call "ad2xy.vi"("DEC"=w2787, "RA"=w2786, "Astrometry"=w2802) -> ("Y"=w2800:dbl, "X"=w2801:dbl)  [unwired: 6 in, 1 out]
                    n5954 = call "ad2xy.vi"("DEC"=w2787, "RA"=w2786, "Astrometry"=w2799) -> ("Y"=w2796:dbl, "X"=w2797:dbl)  [unwired: 6 in, 1 out]
                    n5955 = To Long Integer(number=w2797) -> (32bit integer=w2795:i32)
                    n5956 = To Long Integer(number=w2796) -> (32bit integer=w2794:i32)
                    n5957 = local read "ImgData"() -> (w2798:sgl[][])
                    n5958 = property on="TableXYPos" class="GraphXY (strict)"("Active Cursor"=u32 0, "Cursor.Cursor X"=w2801, "Cursor.Cursor Y"=w2800) -> ()  [unwired: 2 in, 2 out]
                    n5959 = call "subimage.vi"("Ysz/2"=100, "Xsz/2"=100, "Yc"=w2794, "Xc"=w2795, "ImgData"=w2798) -> ("SubImg"=w2782:sgl[][])  [unwired: 6 in]
                    n5960 = local write "SubIMG4DSS?"(TRUE ("SubIMG4DSS?")) -> ()
                    n5961 = Array Max & Min(array=w2782) -> (max value=w2783:sgl)  [unwired: 3 out]
                    n5962 = call "Draw_crosshair.vi"("Image IN"=w2782, "White Value"=w2783) -> ("Image OUT"=w2781:sgl[][])  [unwired: 13 in]
                    n5963 = local write "ImageUsage"(w2778) -> ()
                    n5964 = local write "subimg"(w2781) -> ()
                  }
                  frame 1 {
                    # "Annuler ..."
                    n5965 = control-ref of="TCS actif"() -> (w2803:refnum<vi>)
                    n5966 = local read "TCS VRN"() -> (w2804:refnum<visa-resource-name>)
                    n5967 = call "EXCOM-CMD.vi"("VRN IN"=w2804, "Bool Refnum"=w2803, "Commande #"=13) -> ("VRN OUT"=w2806:refnum<visa-resource-name>, "Error OUT"=w2807:errorcluster)  [unwired: 10 in, 1 out]
                    n5968 = local write "TCS Error"(w2807) -> ()
                    n5969 = local write "TCS VRN"(w2806) -> ()
                  }
                  frame 2 {
                    w2808 = u16 1 items=["Region d'intérêt", "Prévisualisation"] ("ImageUsage")
                    # "Les variables globales servent\npour l'éxécution de starast.vi\n(reste à confirmer l'époque)"
                    # "Devrait probablement vérifier la disponibilité de l'image d'abord."
                    # "Synchroniser la Cible"
                    n5970 = call "ad2deg.vi"("DEC (sec)"=w2822, "RA (sec)"=w2821) -> ("DEC (°)"=w2814:dbl, "RA (°)"=w2815:dbl)
                    n5971 = global write "Globals.vi" "RA Tmp"(w2821) -> ()
                    n5972 = global write "Globals.vi" "DEC Tmp"(w2822) -> ()
                    n5973 = call "precess.vi"("Eq2"=w2813, "Eq1"=w2812, "DEC 1"=w2814, "RA 1"=w2815) -> ("DEC 2"=w2810:dbl, "RA 2"=w2811:dbl)
                    n5974 = local read "ImgAstrom"() -> (w2833:T4)
                    n5975 = local read "FieldAstrom"() -> (w2834:T4)
                    n5976 = call "ad2xy.vi"("DEC"=w2810, "RA"=w2811, "Astrometry"=w2833) -> ("Y"=w2830:dbl, "X"=w2831:dbl)  [unwired: 6 in, 1 out]
                    n5977 = call "ad2xy.vi"("DEC"=w2810, "RA"=w2811, "Astrometry"=w2834) -> ("Y"=w2816:dbl, "X"=w2817:dbl)  [unwired: 6 in, 1 out]
                    n5978 = To Long Integer(number=w2831) -> (32bit integer=w2829:i32)
                    n5979 = To Long Integer(number=w2830) -> (32bit integer=w2828:i32)
                    n5980 = local read "ImgData"() -> (w2832:sgl[][])
                    n5981 = property on="TableXYPos" class="GraphXY (strict)"("Active Cursor"=u32 0, "Cursor.Cursor Position:Cursor X"=w2817, "Cursor.Cursor Position:Cursor Y"=w2816) -> ()  [unwired: 2 in, 2 out]
                    n5982 = call "subimage.vi"("Ysz/2"=100, "Xsz/2"=100, "Yc"=w2828, "Xc"=w2829, "ImgData"=w2832) -> ("SubImg"=w2824:sgl[][])  [unwired: 6 in]
